vi "Instr_InitObject.vi"(8 "error in (no error)":errorcluster, 9 "Instrument Configuration":variant, 10 "GPIB Address":string, 11 "WK6440B in":refnum<class "WK6440B.lvclass">) -> (0 "error out":errorcluster, 3 "WK6440B out":refnum<class "WK6440B.lvclass">)   [LabVIEW 2019, in "WK6440B.lvclass"]
uses:
  WK6440B.lvclass
  InstrumentSetup.vi
  WK6440B_CommandsGlobal.vi
  LCRControl.lvclass
  InstrControl.lvclass
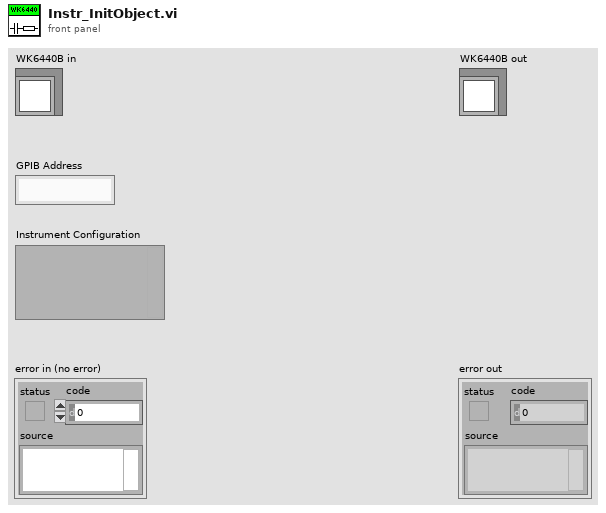
[diagram p1: front panel]
types:
  T1 = cluster{"RC Configuration":u16, "AC amplitude [V]":dbl, "AC frequency [Hz]":i32, "WK6440B":refnum<class "WK6440B.lvclass">}
  T2 = cluster{"Instrument name":string, "Instrument type":u16, "Command \"Initialise LCR\"":string, "Command \"OC Trim\"":string, "Command \"LCR Readout\"":string}
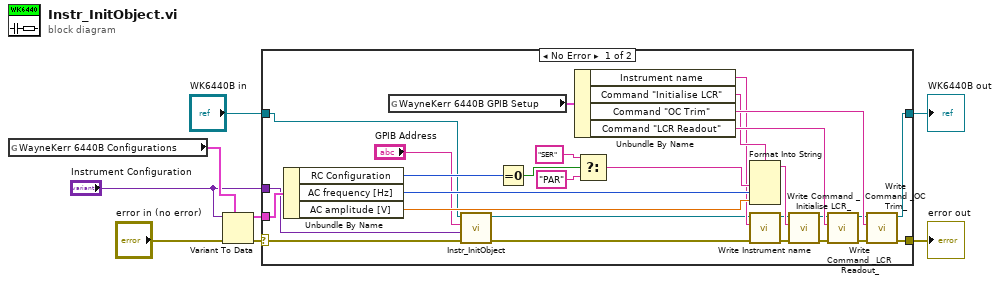
[diagram p0: block diagram]
diagram:
  n1 = global read "InstrumentSetup.vi" "WayneKerr 6440B Configurations"() -> (w4:T1)
  n2 = Variant To Data(error in="error in (no error)", type=w4, Variant="Instrument Configuration") -> (data=w3:T1, error out=w1:errorcluster)
  n3 = case shown="No Error" w1 {
    selector: w1 -> [w17 w38]
    tunnel: [w30 w38] -> w8
    tunnel: [w31 w37] -> w6
    tunnel: "WK6440B in" -> [w18 w37]
    tunnel: w3 -> [w10 _]
    tunnel: "Instrument Configuration" -> [w9 _]
    frame No Error {
      n4 = Unbundle By Name(w10) -> ("RC Configuration"=w27:u16, "AC frequency [Hz]"=w22:i32, "AC amplitude [V]"=w21:dbl)
      n5 = global read "WK6440B_CommandsGlobal.vi" "WayneKerr 6440B GPIB Setup"() -> (w36:T2)
      n6 = call-parent "Instr_InitObject.vi"("error in (no error)"=w17, "Instrument Configuration"=w9, "GPIB Address"="GPIB Address", "LCRControl in"=w18) -> ("error out"=w14:errorcluster, "LCRControl out"=w12:refnum<class "WK6440B.lvclass">)  [unwired: 6 in]
      n7 = Equal To 0?(x=w27) -> (x = 0?=w26:bool)
      n8 = Unbundle By Name(w36) -> ("Instrument name"=w16:string, "Command \"Initialise LCR\""=w20:string, "Command \"OC Trim\""=w34:string, "Command \"LCR Readout\""=w35:string)
      n9 = Select(t="SER", s=w26, f="PAR") -> (s? t:f=w23:string)
      n10 = Format Into String(format string=w20, w23, w22, w21) -> (resulting string=w19:string)  [unwired: 2 in, 1 out]
      n11 = call-dynamic "Write Instrument name.vi"("error in (no error)"=w14, "Instrument name"=w16, "InstControl in"=w12) -> ("error out"=w13:errorcluster, "InstControl out"=w11:refnum<class "WK6440B.lvclass">)  [unwired: 7 in]
      n12 = call-dynamic "Write Command _Initialise LCR_.vi"("error in (no error)"=w13, "Command \"Initialise LCR\""=w19, "LCRControl in"=w11) -> ("error out"=w29:errorcluster, "LCRControl out"=w33:refnum<class "WK6440B.lvclass">)  [unwired: 7 in]
      n13 = call-dynamic "Write Command _LCR Readout_.vi"("error in (no error)"=w29, "Command \"LCR Readout\""=w35, "LCRControl in"=w33) -> ("error out"=w28:errorcluster, "LCRControl out"=w32:refnum<class "WK6440B.lvclass">)  [unwired: 7 in]
      n14 = call-dynamic "Write Command _OC Trim_.vi"("error in (no error)"=w28, "Command \"OC Trim\""=w34, "LCRControl in"=w32) -> ("error out"=w30:errorcluster, "LCRControl out"=w31:refnum<class "WK6440B.lvclass">)  [unwired: 7 in]
    }
    frame Error {
    }
  }
  "error out" <- w8
  "WK6440B out" <- w6
